vi "Format Commands to Tree.vi"(8 "Paths":path[](array[path])=[path "C:/Users/gam.AMER/Documents/2468 code/trunk/FRC/2019/Software/2019 robot/Drive/Commands/Drive for Time.vi", path "C:/Users/gam.AMER/Documents/2468 code/trunk/FRC/2019/Software/2019 robot/Drive/Commands/Drive Immediate.vi", path "C:/Users/gam.AMER/Documents/2468 code/trunk/FRC/2019/Software/2019 robot/Drive/Commands/J-Turn.vi", path "C:/Users/gam.AMER/Documents/2468 code/trunk/FRC/2019/Software/2019 robot/Drive/Commands/Play Path.vi", path "C:/Users/gam.AMER/Documents/2468 code/trunk/FRC/2019/Software/2019 robot/Drive/Commands/Read Drive Operation.vi", path "C:/Users/gam.AMER/Documents/2468 code/trunk/FRC/2019/Software/2019 robot/Drive/Commands/Reserve Drive.vi", path "C:/Users/gam.AMER/Documents/2468 code/trunk/FRC/2019/Software/2019 robot/Drive/Commands/Stop Driving.vi", path "C:/Users/gam.AMER/Documents/2468 code/trunk/FRC/2019/Software/2019 robot/Drive/Commands/Template for Drive Immediate with Deadband.vit", path "C:/Users/gam.AMER/Documents/2468 code/trunk/FRC/2019/Software/2019 robot/Drive/Commands/Template for Drive Immediate.vit", path "C:/Users/gam.AMER/Documents/2468 code/trunk/FRC/2019/Software/2019 robot/Drive/Commands/Template for Drive with Duration.vit", path "C:/Users/gam.AMER/Documents/2468 code/trunk/FRC/2019/Software/2019 robot/Climb/Commands/climb.vi", path "C:/Users/gam.AMER/Documents/2468 code/trunk/FRC/2019/Software/2019 robot/Climb/Commands/Read Climb Operation.vi", path "C:/Users/gam.AMER/Documents/2468 code/trunk/FRC/2019/Software/2019 robot/Climb/Commands/Reserve Climb.vi", path "C:/Users/gam.AMER/Documents/2468 code/trunk/FRC/2019/Software/2019 robot/Climb/Commands/Template for Climb Immediate with Deadband.vit", path "C:/Users/gam.AMER/Documents/2468 code/trunk/FRC/2019/Software/2019 robot/Climb/Commands/Template for Climb Immediate.vit", path "C:/Users/gam.AMER/Documents/2468 code/trunk/FRC/2019/Software/2019 robot/Climb/Commands/Template for Climb with Duration.vit", path "C:/Users/gam.AMER/Documents/2468 code/trunk/FRC/2019/Software/2019 robot/Elevator/Commands/Elevator Immediate.vi", path "C:/Users/gam.AMER/Documents/2468 code/trunk/FRC/2019/Software/2019 robot/Elevator/Commands/Read Elevator Operation.vi", path "C:/Users/gam.AMER/Documents/2468 code/trunk/FRC/2019/Software/2019 robot/Elevator/Commands/Reserve Elevator.vi", path "C:/Users/gam.AMER/Documents/2468 code/trunk/FRC/2019/Software/2019 robot/Elevator/Commands/Template for Elevator Immediate with Deadband.vit", path "C:/Users/gam.AMER/Documents/2468 code/trunk/FRC/2019/Software/2019 robot/Elevator/Commands/Template for Elevator Immediate.vit", path "C:/Users/gam.AMER/Documents/2468 code/trunk/FRC/2019/Software/2019 robot/Elevator/Commands/Template for Elevator with Duration.vit", path "C:/Users/gam.AMER/Documents/2468 code/trunk/FRC/2019/Software/2019 robot/Floating Intake/Commands/Duration Intake.vi", path "C:/Users/gam.AMER/Documents/2468 code/trunk/FRC/2019/Software/2019 robot/Floating Intake/Commands/Floating Intake Immediate.vi", path "C:/Users/gam.AMER/Documents/2468 code/trunk/FRC/2019/Software/2019 robot/Floating Intake/Commands/Floating Intake Read.vi", path "C:/Users/gam.AMER/Documents/2468 code/trunk/FRC/2019/Software/2019 robot/Floating Intake/Commands/Read Floating Intake Operation.vi", path "C:/Users/gam.AMER/Documents/2468 code/trunk/FRC/2019/Software/2019 robot/Floating Intake/Commands/Reserve Floating Intake.vi", path "C:/Users/gam.AMER/Documents/2468 code/trunk/FRC/2019/Software/2019 robot/Floating Intake/Commands/Template for Floating Intake Immediate with Deadband.vit", path "C:/Users/gam.AMER/Documents/2468 code/trunk/FRC/2019/Software/2019 robot/Floating Intake/Commands/Template for Floating Intake Immediate.vit", path "C:/Users/gam.AMER/Documents/2468 code/trunk/FRC/2019/Software/2019 robot/Floating Intake/Commands/Template for Floating Intake with Duration.vit", path "C:/Users/gam.AMER/Documents/2468 code/trunk/FRC/2019/Software/2019 robot/Carriage Intake/Commands/Carriage Intake Immediate with Deadband.vi", path "C:/Users/gam.AMER/Documents/2468 code/trunk/FRC/2019/Software/2019 robot/Carriage Intake/Commands/Carriage Intake Immediate.vi", path "C:/Users/gam.AMER/Documents/2468 code/trunk/FRC/2019/Software/2019 robot/Carriage Intake/Commands/Read Carriage Intake Operation.vi", path "C:/Users/gam.AMER/Documents/2468 code/trunk/FRC/2019/Software/2019 robot/Carriage Intake/Commands/Reserve Carriage Intake.vi", path "C:/Users/gam.AMER/Documents/2468 code/trunk/FRC/2019/Software/2019 robot/Carriage Intake/Commands/Template for Carriage Intake Immediate with Deadband.vit", path "C:/Users/gam.AMER/Documents/2468 code/trunk/FRC/2019/Software/2019 robot/Carriage Intake/Commands/Template for Carriage Intake Immediate.vit", path "C:/Users/gam.AMER/Documents/2468 code/trunk/FRC/2019/Software/2019 robot/Carriage Intake/Commands/Template for Carriage Intake with Duration.vit", path "C:/Users/gam.AMER/Documents/2468 code/trunk/FRC/2019/Software/2019 robot/LattePanda/Commands/Is Connected.vi", path "C:/Users/gam.AMER/Documents/2468 code/trunk/FRC/2019/Software/2019 robot/LattePanda/Commands/Power On.vi", path "C:/Users/gam.AMER/Documents/2468 code/trunk/FRC/2019/Software/2019 robot/LattePanda/Commands/Read LattePanda Operation.vi", path "C:/Users/gam.AMER/Documents/2468 code/trunk/FRC/2019/Software/2019 robot/LattePanda/Commands/Reserve LattePanda.vi", path "C:/Users/gam.AMER/Documents/2468 code/trunk/FRC/2019/Software/2019 robot/LattePanda/Commands/Shut Down.vi", path "C:/Users/gam.AMER/Documents/2468 code/trunk/FRC/2019/Software/2019 robot/LattePanda/Commands/Template for LattePanda Immediate with Deadband.vit", path "C:/Users/gam.AMER/Documents/2468 code/trunk/FRC/2019/Software/2019 robot/LattePanda/Commands/Template for LattePanda Immediate.vit", path "C:/Users/gam.AMER/Documents/2468 code/trunk/FRC/2019/Software/2019 robot/LattePanda/Commands/Template for LattePanda with Duration.vit"], 9 "Command Info":T4(array[cluster]), 11 "Tree Refnum":refnum<vi>) -> (2 "2D Picture":picture, 3 "Filtered Command Info Out":T1)   [LabVIEW 2025]
uses:
  <vilib>/picture/picture.llb/imagedata.ctl
  Types/Command Editor Info.ctl
  Types/Single Cmd Info.ctl
  <vilib>/Utility/Data Type/NI_Data Type.lvlib
panel:
  in  "Tree":string(tree)
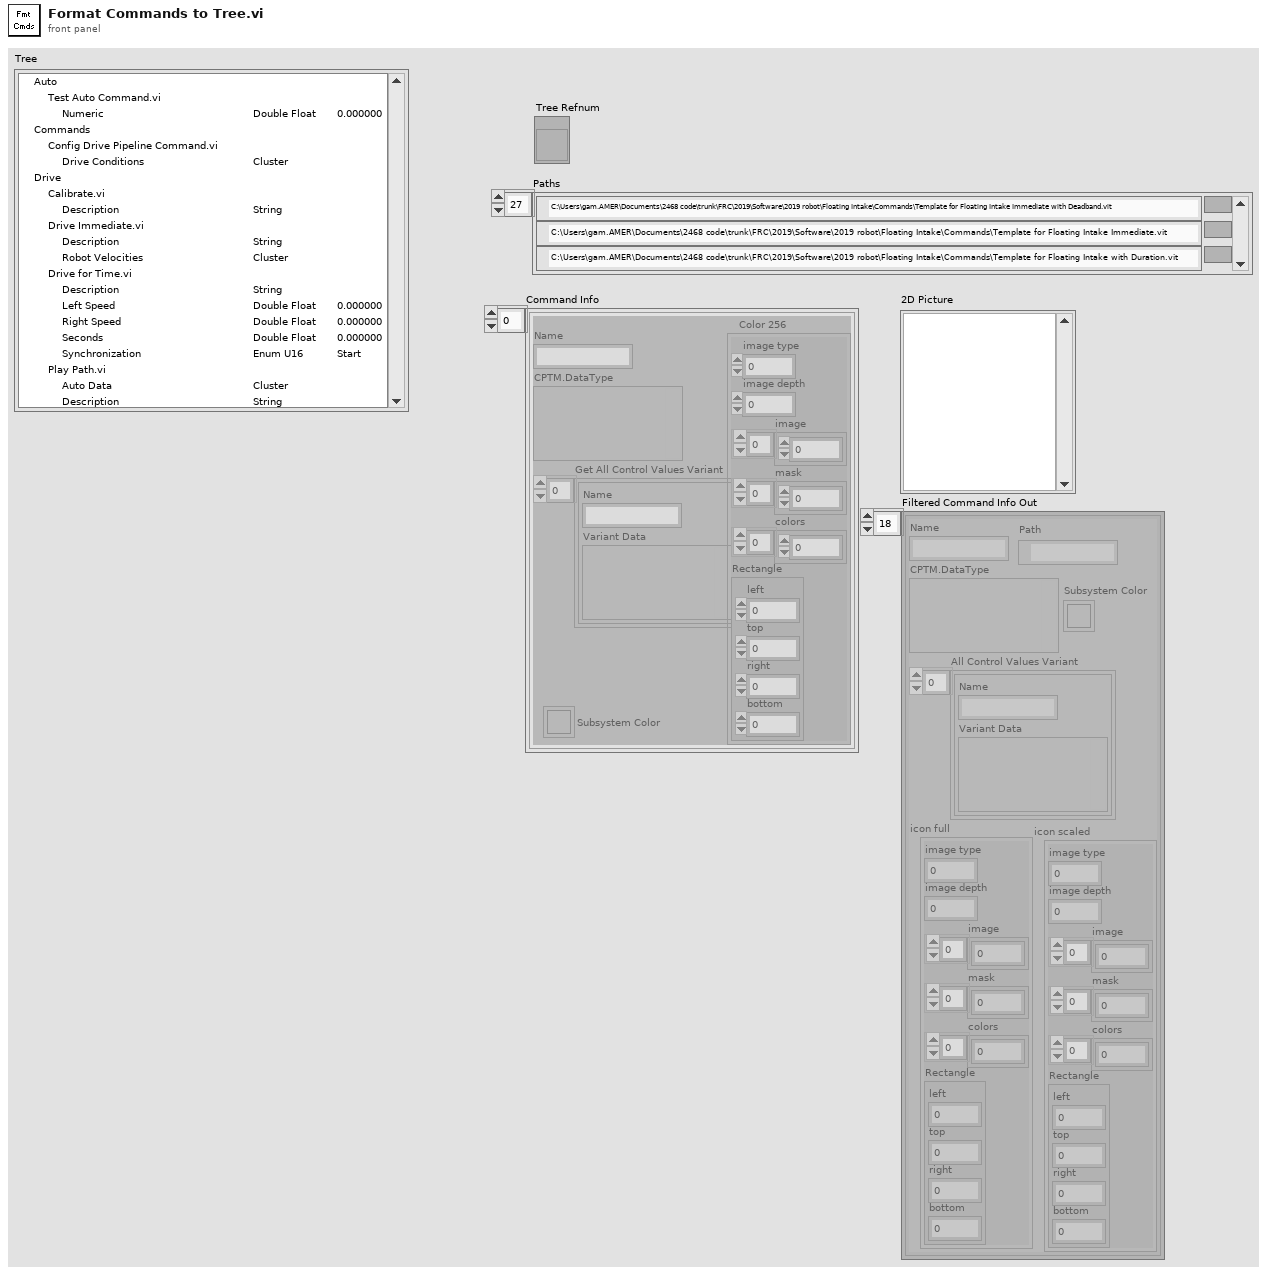
[diagram p1: front panel]
types:
  T1 = typedef "Command Editor Info.ctl" = T2[]
  T2 = typedef "Single Cmd Info.ctl" = cluster{"Name":string, "CPTM.DataType":variant, "All Control Values Variant":cluster{"Name":string, "Variant Data":variant}[], "icon full":T3, "icon scaled":T3, "Path":path, "Subsystem Color":u32}
  T3 = typedef "imagedata.ctl" = cluster{"image type":i32, "image depth":i32, "image":u8[], "mask":u8[], "colors":u32[], "Rectangle":cluster{"left":i16, "top":i16, "right":i16, "bottom":i16}}
  T4 = cluster{"Name":string, "CPTM.DataType":variant, "Get All Control Values Variant":cluster{"Name":string, "Variant Data":variant}[], "Color 256":T3, "Subsystem Color":u32}[]
  T5 = cluster{"Left Cell String":string, "Child Text":string[], "Child Tag":string, "Item Indent":i32, "Child Only?":bool, "Glyph Index":i32}
  T6 = cluster{"Left Cell String":string, "Child Text":string[], "Child Tag":string, "Item Indent":i32, "Child Only?":bool, "Glyph Index":i32}[]
  T7 = cluster{"Name":string, "CPTM.DataType":variant, "Get All Control Values Variant":cluster{"Name":string, "Variant Data":variant}[], "Color 256":T3, "Color 256":T3, "Path":path, "Subsystem Color":u32}
  T8 = typedef "NI_Data Type.lvlib/Data Type.ctl" = enum8{"Invalid Type", "Void", "I8", "I16", "I32", "I64", "U8", "U16", "U32", "U64", "Single Float", "Double Float", "Extended Float", "Single Complex", "Double Complex", "Extended Complex", "Enum U8", "Enum U16", "Enum U32", "Enum U64", "Single Float With Unit", "Double Float With Unit", "Extended Float With Unit", "Single Complex with Unit", "Double Complex with Unit", "Extended Complex with Unit", "Boolean", "String", "Path", "Picture", "Tag", "Array", "Cluster", "Variant", "LV Variant", "Waveform", "Timestamp", "Digital Waveform", "Digital Data", "ExpressData", "Refnum", "External Data", "VI", "Poly VI", "LabVIEW Class Instance", "Fixed Point", "Set Collection", "Map Collection"}
  T9 = typedef "NI_Data Type.lvlib/Type Definition Info.ctl" = cluster{"Name":string, "Timestamp":u32}
  T10 = cluster{"left":i16, "top":i16, "right":i16, "bottom":i16}
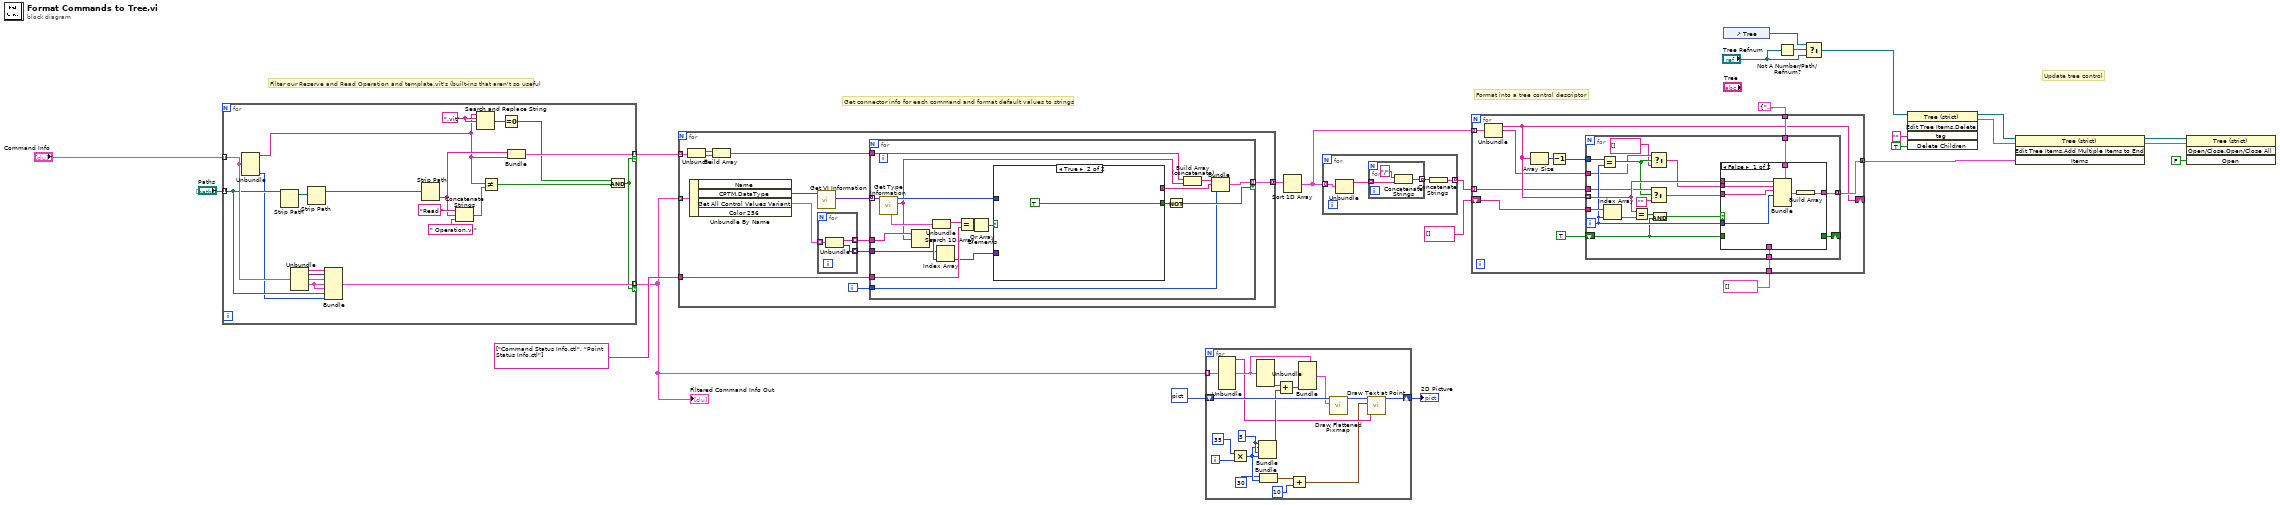
[diagram p0: block diagram]
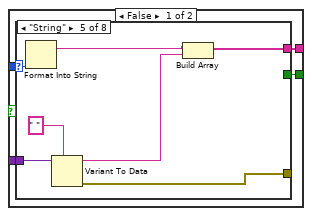
[diagram p2: hidden frame]
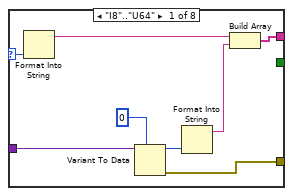
[diagram p3: hidden frame]
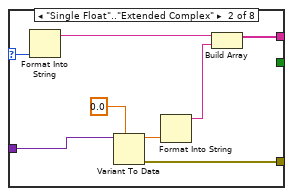
[diagram p4: hidden frame]
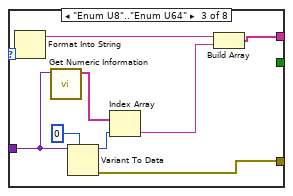
[diagram p5: hidden frame]
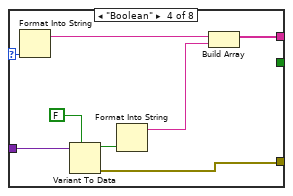
[diagram p6: hidden frame]
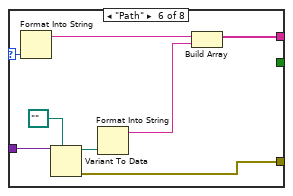
[diagram p7: hidden frame]
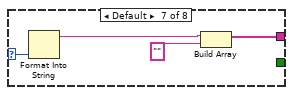
[diagram p8: hidden frame]
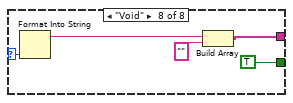
[diagram p9: hidden frame]
diagram:
  # "Update tree control"
  # "Get connector info for each command and format default values to strings"
  # "Filter our Reserve and Read Operation and template.vit's (built-ins that aren't so useful"
  # "Format into a tree control descriptor"
  n1 = for {
    tunnel: "Command Info" -> [w36] mode=indexing
    tunnel: "Paths" -> [w35] mode=indexing
    tunnel: [w44] -> w3 mode=indexing if=w28
    tunnel: [w37] -> w2 mode=indexing if=w28
    w33 = ".vit" ("search string")
    n2 = Unbundle(w36) -> ("Name"=w26:string, "Subsystem Color"=w34:u32)  [unwired: 3 out]
    n3 = Strip Path(path=w35) -> (stripped path=w46:path)  [unwired: 1 out]
    n4 = Unbundle(w36) -> ("Name"=w38:string, "CPTM.DataType"=w39:variant, "Get All Control Values Variant"=w40:cluster{"Name":string, "Variant Data":variant}[], "Color 256"=w41:T3)  [unwired: 1 out]
    n5 = Strip Path(path=w46) -> (stripped path=w45:path)  [unwired: 1 out]
    n6 = Bundle("Name"=w38, "CPTM.DataType"=w39, "Get All Control Values Variant"=w40, "Color 256"=w41, "Color 256"=w41, "Path"=w35, "Subsystem Color"=w34) -> (w37:T7)  [unwired: 1 in]
    n7 = Strip Path(path=w45) -> (name=w27:string)  [unwired: 1 out]
    n8 = Concatenate Strings("Read ", w27, " Operation.vi") -> (w30:string)
    n9 = Search and Replace String(input string=w26, search string=w33, replace string=w33) -> (number of replacements=w32:i32)  [unwired: 5 in, 3 out]
    n10 = Not Equal?(x=w26, y=w30) -> (x != y?=w29:bool)
    n11 = Equal To 0?(x=w32) -> (x = 0?=w31:bool)
    n12 = Bundle("name"=w27, "Name"=w26) -> (w44:cluster{"name":string, "Name":string})  [unwired: 1 in]
    n13 = Compound Arithmetic op=AND(w31, w29) -> (w28:bool)
  }
  "Filtered Command Info Out" <- w2
  n14 = for {
    tunnel: w3 -> [w59] mode=indexing
    tunnel: [w52] -> w22 mode=concatenating
    tunnel: w2 -> [w56] mode=indexing
    tunnel: string[] ["Command Status Info.ctl", "Point Status Info.ctl"] ("Name") -> [w51]
    i -> [w47]
    n15 = Unbundle(w59) -> ("name"=w58:string, "Name"=w57:string)
    n16 = Unbundle By Name(w56) -> ("CPTM.DataType"=w55:variant, "Get All Control Values Variant"=w50:cluster{"Name":string, "Variant Data":variant}[])  [unwired: 2 out]
    n17 = Build Array(w58, w57) -> (w54:string[])
    n18 = call <vilib>:"Get VI Information.vi"("variant"=w55) -> ("VI terminal types"=w53:variant[])  [unwired: 7 in, 3 out]
    n19 = for {
      tunnel: w50 -> [w62] mode=indexing
      tunnel: [w61] -> w49 mode=indexing
      tunnel: [w60] -> w48 mode=indexing
      n20 = Unbundle(w62) -> ("Name"=w61:string, "Variant Data"=w60:variant)
    }
    n21 = for {
      tunnel: w54 -> [w79]
      tunnel: w53 -> [w81] mode=indexing
      tunnel: [w77] -> w52 mode=indexing if=w72
      tunnel: w51 -> [w75]
      tunnel: w49 -> [w70]
      tunnel: w48 -> [w67]
      tunnel: w47 -> [w65]
      n22 = call <vilib>:"Get Type Information.vi"("variant"=w81) -> ("name"=w69:string, "type"=w80:T8, "type definition info"=w76:T9)  [unwired: 6 in, 2 out]
      n23 = Search 1D Array(1D array=w70, element=w69) -> (index of element=w68:i32)  [unwired: 1 in]
      n24 = Unbundle(w76) -> ("Name"=w74:string)  [unwired: 1 out]
      n25 = Index Array(array=w67, index=w68) -> (element=w66:variant)
      n26 = Equal?(x=w74, y=w75) -> (x = y?=w64:bool[])
      n27 = Or Array Elements(Boolean array=w64) -> (logical OR=w63:bool)
      n28 = case shown="True" w63 {
        tunnel: w80 -> [w85 _]
        tunnel: [w84 _] -> w71
        tunnel: [w83 TRUE] -> w73
        tunnel: w66 -> [w82 _]
        frame False {
          n29 = case shown="\"String\"" w85 {
            selector: w85 -> [w93 w101 w110 w118 w125 w133 w137 w142]
            tunnel: [w88 w95 w107 w113 w122 w128 w135 w139] -> w84
            tunnel: [_ _ _ _ _ _ _ TRUE] -> w83
            tunnel: w82 -> [w87 w98 w105 w115 w124 w130 _ _]
            tunnel: [w86 w94 w106 w111 w119 w126 _ _] -> _
            frame "I8".."U64" {
              n30 = Format Into String(w93) -> (resulting string=w89:string)  [unwired: 3 in, 1 out]
              n31 = Variant To Data(type=i64 0, Variant=w87) -> (data=w91:i64, error out=w86:errorcluster)  [unwired: 1 in]
              n32 = Format Into String(w91) -> (resulting string=w90:string)  [unwired: 3 in, 1 out]
              n33 = Build Array(w89, w90) -> (w88:string[])
            }
            frame "Single Float".."Extended Complex" {
              n34 = Format Into String(w101) -> (resulting string=w97:string)  [unwired: 3 in, 1 out]
              n35 = Variant To Data(type=0.0, Variant=w98) -> (data=w99:dbl, error out=w94:errorcluster)  [unwired: 1 in]
              n36 = Format Into String(w99) -> (resulting string=w96:string)  [unwired: 3 in, 1 out]
              n37 = Build Array(w97, w96) -> (w95:string[])
            }
            frame "Enum U8".."Enum U64" {
              n38 = Format Into String(w110) -> (resulting string=w108:string)  [unwired: 3 in, 1 out]
              n39 = call <vilib>:"Get Numeric Information.vi"("variant"=w105) -> ("enum names"=w104:string[])  [unwired: 7 in, 3 out]
              n40 = Variant To Data(type=i64 0, Variant=w105) -> (data=w103:i64, error out=w106:errorcluster)  [unwired: 1 in]
              n41 = Index Array(array=w104, index=w103) -> (element=w102:string)
              n42 = Build Array(w108, w102) -> (w107:string[])
            }
            frame "Boolean" {
              n43 = Format Into String(w118) -> (resulting string=w114:string)  [unwired: 3 in, 1 out]
              n44 = Variant To Data(type=FALSE, Variant=w115) -> (data=w116:bool, error out=w111:errorcluster)  [unwired: 1 in]
              n45 = Format Into String(w116) -> (resulting string=w112:string)  [unwired: 3 in, 1 out]
              n46 = Build Array(w114, w112) -> (w113:string[])
            }
            frame "String" {
              n47 = Format Into String(w125) -> (resulting string=w123:string)  [unwired: 3 in, 1 out]
              n48 = Variant To Data(type=" ", Variant=w124) -> (data=w121:string, error out=w119:errorcluster)  [unwired: 1 in]
              n49 = Build Array(w123, w121) -> (w122:string[])
            }
            frame "Path" {
              n50 = Format Into String(w133) -> (resulting string=w129:string)  [unwired: 3 in, 1 out]
              n51 = Variant To Data(type=path "", Variant=w130) -> (data=w131:path, error out=w126:errorcluster)  [unwired: 1 in]
              n52 = Format Into String(w131) -> (resulting string=w127:string)  [unwired: 3 in, 1 out]
              n53 = Build Array(w129, w127) -> (w128:string[])
            }
            frame Default {
              n54 = Format Into String(w137) -> (resulting string=w136:string)  [unwired: 3 in, 1 out]
              n55 = Build Array(w136, "") -> (w135:string[])
            }
            frame "Void" {
              n56 = Format Into String(w142) -> (resulting string=w140:string)  [unwired: 3 in, 1 out]
              n57 = Build Array(w140, "") -> (w139:string[])
            }
          }
        }
        frame True {
        }
      }
      n58 = Not(x=w73) -> (.not. x?=w72:bool)
      n59 = Build Array (concatenate)(w79, w69) -> (w78:string[])
      n60 = Bundle(w78, w71, w65) -> (w77:cluster{string[], string[], i32})  [unwired: 1 in]
    }
  }
  n61 = for {
    tunnel: w2 -> [w160] mode=indexing
    shift-right: [w151] -> w4
    shift-left: picture data[5B] ("2D Picture") -> [w161]
    i -> [w156]
    w155 = 5
    n62 = Unbundle(w160) -> ("Name"=w147:string, "Color 256"=w159:T3)  [unwired: 5 out]
    n63 = Multiply(x=35, y=w156) -> (x*y=w149:i32)
    n64 = Unbundle(w159) -> ("Rectangle"=w157:T10)  [unwired: 5 out]
    n65 = Bundle(w155, w149, w155, w149) -> (w154:cluster{i32, i32, i32, i32})  [unwired: 1 in]
    n66 = Bundle(30, w149) -> (w146:cluster{i32, i32})  [unwired: 1 in]
    n67 = Add(x=w157, y=w154) -> (x+y=w153:cluster{i32, i32, i32, i32})
    n68 = Add(x=w146, y=10) -> (x+y=w145:cluster{i32, i32})
    n69 = Bundle(cluster=w159, "Rectangle"=w153) -> (w158:T3)  [unwired: 5 in]
    n70 = call <vilib>:"Draw Flattened Pixmap.vi"("image data"=w158, "picture"=w161) -> ("new picture"=w152:picture)  [unwired: 7 in]
    n71 = call <vilib>:"Draw Text at Point.vi"("text"=w147, "origin"=w145, "picture"=w152) -> ("new picture"=w151:picture)  [unwired: 7 in, 1 out]
  }
  "2D Picture" <- w4
  n72 = Sort 1D Array(array=w22) -> (sorted array=w23:cluster{string[], string[], i32}[])
  n73 = for {
    tunnel: w23 -> [w165] mode=indexing
    tunnel: [w162] -> w24 mode=indexing
    n74 = Unbundle(w165) -> (w164:string[])  [unwired: 2 out]
    n75 = for {
      tunnel: w164 -> [w167] mode=indexing
      tunnel: [w166] -> w163 mode=indexing
      n76 = Concatenate Strings("/", w167) -> (w166:string)
    }
    n77 = Concatenate Strings(w163) -> (w162:string)
  }
  n78 = for {
    tunnel: [w175] -> w25 mode=concatenating
    tunnel: T5 {"Left Cell String"="", "Child Text"=[], "Child Tag"="", "Item Indent"=0, "Child Only?"=FALSE, "Glyph Index"=0} ("Item") -> [w176]
    shift-right: [w172] -> _
    shift-left: string[] [] ("Child Text") -> [w178]
    tunnel: w23 -> [w179] mode=indexing
    tunnel: T6 [] -> [w177]
    tunnel: w24 -> [w171] mode=indexing
    n79 = Unbundle(w179) -> (w172:string[], w169:string[])  [unwired: 1 out]
    n80 = Array Size(array=w172) -> (size(s)=w174:i32)
    n81 = Decrement(x=w174) -> (x-1=w173:i32)
    n82 = for {
      tunnel: w178 -> [w198]
      tunnel: w172 -> [w193] mode=indexing
      tunnel: w177 -> [w196]
      tunnel: [w195] -> w175 mode=concatenating
      tunnel: w176 -> [w194]
      tunnel: w173 -> [w191]
      tunnel: w169 -> [w181]
      tunnel: w171 -> [w189]
      shift-right: [w185] -> _
      shift-left: TRUE -> [w184]
      i -> [w192]
      n83 = Equal?(x=w191, y=w192) -> (x = y?=w182:bool)
      n84 = Index Array(array=w198, index=w192) -> (element=w197:string)
      n85 = Equal?(x=w193, y=w197) -> (x = y?=w187:bool)
      n86 = Select(t=w189, s=w182, f="") -> (s? t:f=w190:string)
      n87 = Select(t=w181, s=w182, f=string[] [] ("appended array")) -> (s? t:f=w183:string[])
      n88 = And(x=w187, y=w184) -> (x .and. y?=w186:bool)
      n89 = case shown="False" w186 {
        tunnel: [w203 w207] -> w195
        tunnel: w196 -> [_ w207]
        tunnel: w194 -> [w205 _]
        tunnel: w193 -> [w202 _]
        tunnel: w192 -> [w201 _]
        tunnel: w183 -> [w200 _]
        tunnel: w190 -> [w199 _]
        tunnel: [_ w206] -> w185
        tunnel: w184 -> [_ w206]
        frame False {
          n90 = Bundle(cluster=w205, "Left Cell String"=w202, "Child Text"=w200, "Child Tag"=w199, "Item Indent"=w201) -> (w204:T5)  [unwired: 2 in]
          n91 = Build Array(w204) -> (w203:T6)
        }
        frame True {
        }
      }
    }
  }
  n92 = control-ref of="Tree"() -> (w7:refnum<vi>)
  n93 = Not A Number/Path/Refnum?(number/path/refnum="Tree Refnum") -> (NaN/Path/Refnum?=w11:bool)
  n94 = Select(t=w7, s=w11, f="Tree Refnum") -> (s? t:f=w10:refnum<vi>)
  n95 = invoke on="Invoke Node" class="Tree (strict)" method="Edit Tree Items.Delete"(reference=w10, "tag"="" ("Tag"), "Delete Children"=TRUE ("Delete Children?")) -> (reference out=w9:refnum<vi>, error out=w16:errorcluster)  [unwired: 2 in, 3 out]
  n96 = invoke on="Invoke Node" class="Tree (strict)" method="Edit Tree Items.Add Multiple Items to End"(reference=w9, error in=w16, "Items"=w25) -> (reference out=w8:refnum<vi>, error out=w13:errorcluster)  [unwired: 1 in, 2 out]
  n97 = invoke on="Invoke Node" class="Tree (strict)" method="Open/Close.Open/Close All"(reference=w8, error in=w13, "Open"=FALSE ("Open?")) -> ()  [unwired: 1 in, 4 out]
